vi "Configure.vi"(8 "error in (no error)":errorcluster, 11 "Waveform in":refnum<class "Waveform.lvclass">) -> (0 "error out":errorcluster, 2 "cancelled?":bool, 3 "Waveform out":refnum<class "Waveform.lvclass">)   [LabVIEW 2012, in "Waveform.lvclass"]
doc: "The configure method configures the details for the RabbitMQ connection, the observers and the mapping script.\n\nIn the derived class, make a call to the parent for setting these parameters."
uses:
  Waveform.lvclass
  <vilib>/Distrio/Murmex/Murmex/Murmex.lvclass
  <vilib>/Utility/miscctls.llb/LVPointTypeDef.ctl
panel:
  in  "button::cancel":bool
  in  "button::ok":bool
  in  "button::configure murmex":bool
  in  "Tab Control":T1(tab)
  in  "Output Terminal 2":tag="/Dev1/PFI12" caption="Output Terminal"
  in  "Counter 2":tag="Dev1/ctr0" caption="Counter"
  in  "Frequency 2":dbl caption="Frequency"
  in  "Duty cycle 2":dbl caption="Duty cycle"
  in  "Output Terminal":tag="/Dev1/PFI12"
  in  "Counter":tag="Dev1/ctr0"
  in  "Frequency":dbl
  in  "Duty cycle":dbl
  in  "Physical Channel 3":tag="Dev1/ao0" caption="Physical Channel"
  in  "min Voltage 3":dbl caption="min Voltage"
  in  "max Voltage 3":dbl caption="max Voltage"
  in  "trigger source 3":tag caption="trigger source"
  in  "trigger edge 3":i32(ring)=10280 caption="trigger edge 2" items=["Rising"=10280, "Falling"=10171]
  in  "Physical Channel 2":tag="Dev1/ao0" caption="Physical Channel"
  in  "min Voltage 2":dbl caption="min Voltage"
  in  "max Voltage 2":dbl caption="max Voltage"
  in  "trigger source 2":tag caption="trigger source"
  in  "trigger edge 2":i32(ring)=10280 items=["Rising"=10280, "Falling"=10171]
  in  "Physical Channel":tag="Dev1/ao0"
  in  "min Voltage":dbl
  in  "max Voltage":dbl
  in  "trigger source":tag
  in  "trigger edge":i32(ring)=10280 items=["Rising"=10280, "Falling"=10171]
  in  "camera 1":string
  in  "camera 2":string
  in  "camera 3":string
  # "RabbitMQ parameters"
  # "Window position"
  # "Sends a setting or configuration value to an observer, e.g. observer.parameter=settingsname;"
  # "Frame counter"
  # "Clock for AO channels"
  # "Galvo 1"
  # "Galvo 2"
  # "Pockels Cell"
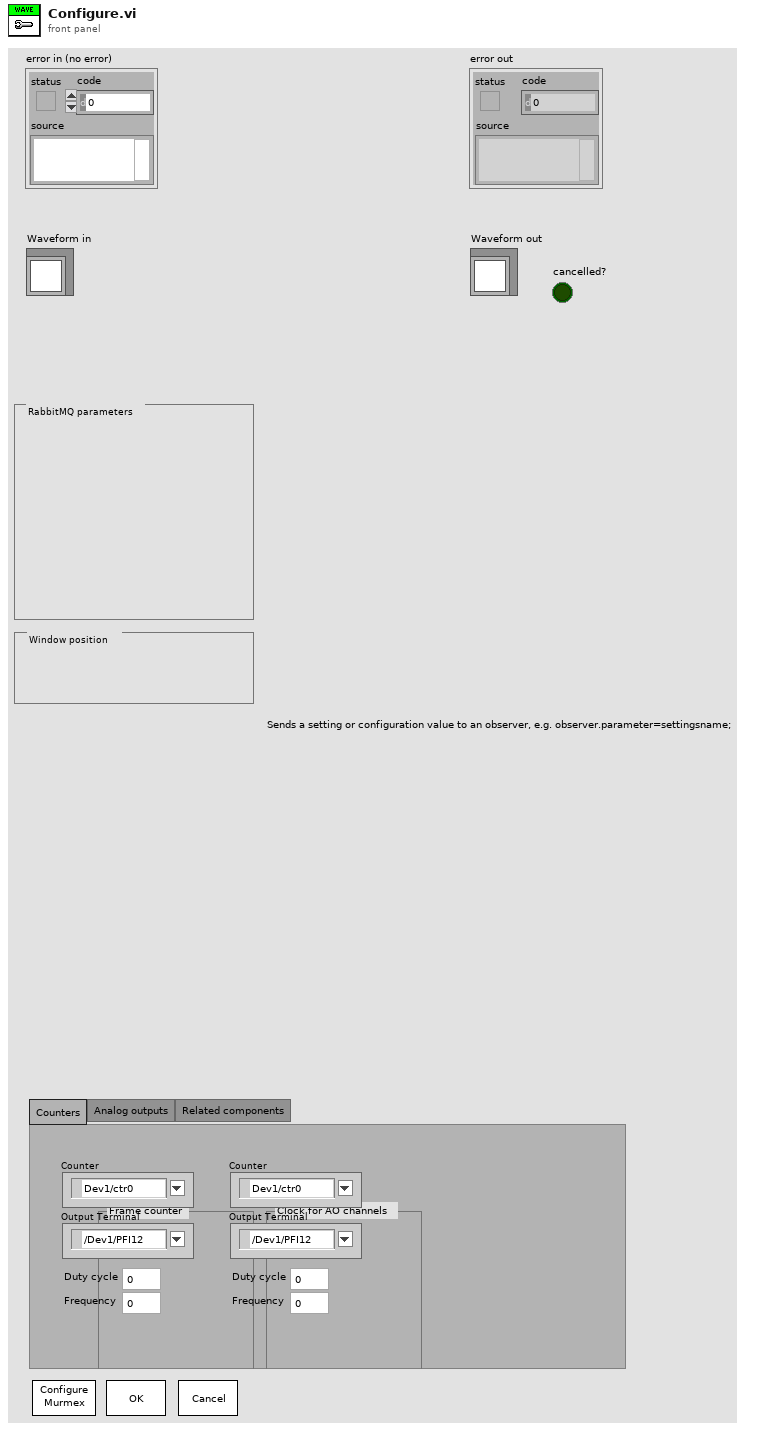
[diagram p1: front panel]
types:
  T1 = enum32{"Counters", "Analog outputs", "Related components"}
  T2 = typedef "LVPointTypeDef.ctl" = cluster{"Horizontal":i16, "Vertical":i16}
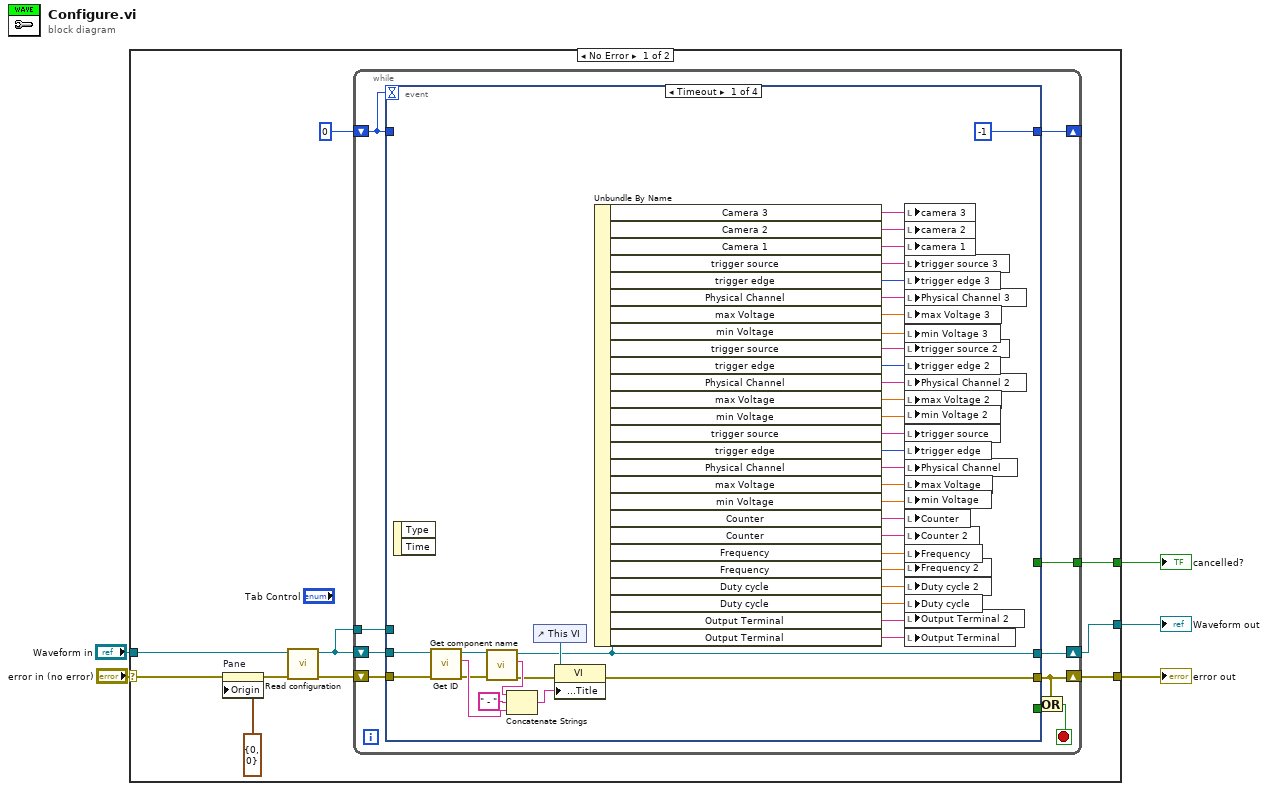
[diagram p0: block diagram]
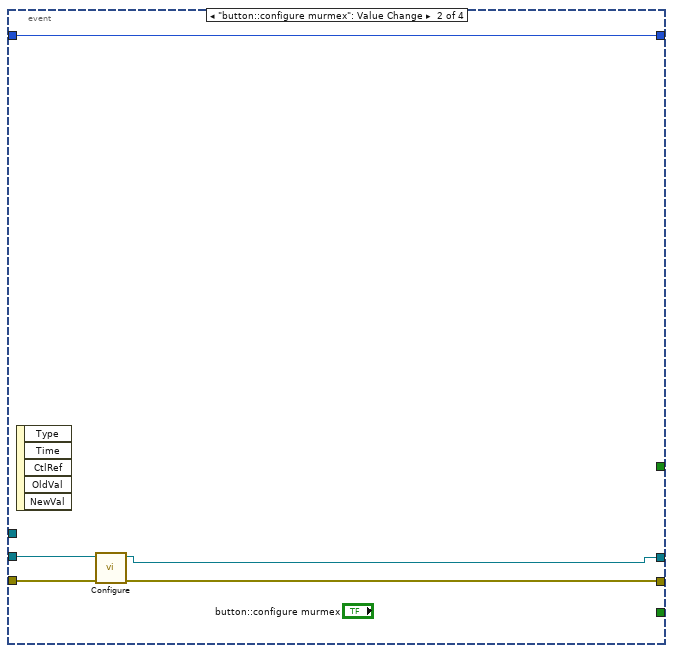
[diagram p2: hidden frame]
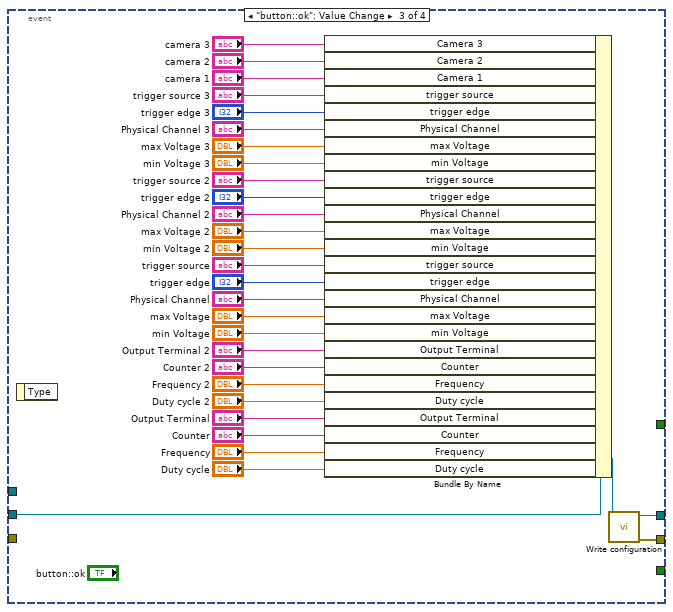
[diagram p3: hidden frame]
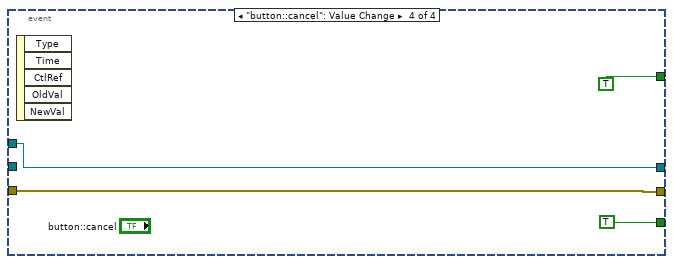
[diagram p4: hidden frame]
diagram:
  n1 = case shown="No Error" "error in (no error)" {
    selector: "error in (no error)" -> [w14 w105]
    tunnel: "Waveform in" -> [w12 w104]
    tunnel: [w8 w105] -> w3
    tunnel: [w7 w104] -> w2
    tunnel: [w6 _] -> w1
    frame No Error {
      n2 = property on="Pane" class="Pane"(error in=w14, "Origin"=T2 {"Horizontal"=0, "Vertical"=0}) -> (error out=w13:errorcluster)  [unwired: 1 in, 1 out]
      n3 = call <vilib>:"Read configuration.vi"("error in (no error)"=w13, "Murmex in"=w12) -> ("error out"=w11:errorcluster, "Murmex out"=w10:refnum<class "Waveform.lvclass">)  [unwired: 7 in, 1 out]
      n4 = while {
        shift-right: [w19] -> w8
        shift-left: w11 -> [w25]
        shift-right: [w21] -> w7
        shift-left: w10 -> [w23]
        tunnel: w10 -> [w24]
        shift-right: [w20] -> _
        shift-left: 0 -> [w22]
        tunnel: [w16] -> w6
        stop <- w18 stop-if-true
        n5 = event shown="[0] Timeout" {
          selector: _ -> [_ _ _ _]
          dyn-events: _ -> [_ _ _ _]
          timeout: w22 -> [_ _ _ _]
          tunnel: w25 -> [w64 w69 _ w103]
          tunnel: w24 -> [_ _ _ w102]
          tunnel: w23 -> [w63 w66 w97 _]
          tunnel: w22 -> [_ w67 _ _]
          tunnel: [w54 w68 w98 w103] -> w19
          tunnel: [w53 w65 w99 w102] -> w21
          tunnel: [-1 w67 _ _] -> w20
          tunnel: [_ _ _ TRUE ("force loading?")] -> w17
          tunnel: [_ _ _ TRUE ("force loading?")] -> w16
          event Timeout {
            n6 = event-data() -> ()  [unwired: 1 in, 2 out]
            n7 = call <vilib>:"Get ID.vi"("error in (no error)"=w64, "Murmex in"=w63) -> ("error out"=w58:errorcluster, "component id"=w61:string, "Murmex out"=w59:refnum<class "Waveform.lvclass">)  [unwired: 7 in]
            n8 = call <vilib>:"Get component name.vi"("error in (no error)"=w58, "Murmex in"=w59) -> ("error out"=w56:errorcluster, "component name"=w60:string, "Murmex out"=w53:refnum<class "Waveform.lvclass">)  [unwired: 7 in]
            n9 = Concatenate Strings(w60, " - " ("string"), w61) -> (w55:string)
            n10 = control-ref of="This VI"() -> (w57:refnum<vi>)
            n11 = property class="VI"(reference=w57, error in=w56, "Front Panel.Title"=w55) -> (error out=w54:errorcluster)  [unwired: 1 out]
            n12 = Unbundle By Name(w53) -> ("Camera 3"=w26:string, "Camera 2"=w27:string, "Camera 1"=w28:string, "trigger source"=w29:tag, "trigger edge"=w30:i32, "Physical Channel"=w31:tag, "max Voltage"=w32:dbl, "min Voltage"=w33:dbl, "trigger source"=w38:tag, "trigger edge"=w37:i32, "Physical Channel"=w36:tag, "max Voltage"=w35:dbl, "min Voltage"=w34:dbl, "trigger source"=w39:tag, "trigger edge"=w40:i32, "Physical Channel"=w41:tag, "max Voltage"=w42:dbl, "min Voltage"=w43:dbl, "Counter"=w46:tag, "Counter"=w47:tag, "Frequency"=w45:dbl, "Frequency"=w44:dbl, "Duty cycle"=w48:dbl, "Duty cycle"=w49:dbl, "Output Terminal"=w51:tag, "Output Terminal"=w50:tag)
            n13 = local write "camera 3"(w26) -> ()
            n14 = local write "camera 2"(w27) -> ()
            n15 = local write "camera 1"(w28) -> ()
            n16 = local write "trigger source 3"(w29) -> ()
            n17 = local write "trigger edge 3"(w30) -> ()
            n18 = local write "Physical Channel 3"(w31) -> ()
            n19 = local write "max Voltage 3"(w32) -> ()
            n20 = local write "min Voltage 3"(w33) -> ()
            n21 = local write "trigger source 2"(w38) -> ()
            n22 = local write "trigger edge 2"(w37) -> ()
            n23 = local write "Physical Channel 2"(w36) -> ()
            n24 = local write "max Voltage 2"(w35) -> ()
            n25 = local write "min Voltage 2"(w34) -> ()
            n26 = local write "trigger source"(w39) -> ()
            n27 = local write "trigger edge"(w40) -> ()
            n28 = local write "Physical Channel"(w41) -> ()
            n29 = local write "max Voltage"(w42) -> ()
            n30 = local write "min Voltage"(w43) -> ()
            n31 = local write "Counter"(w46) -> ()
            n32 = local write "Counter 2"(w47) -> ()
            n33 = local write "Frequency"(w45) -> ()
            n34 = local write "Frequency 2"(w44) -> ()
            n35 = local write "Duty cycle 2"(w48) -> ()
            n36 = local write "Duty cycle"(w49) -> ()
            n37 = local write "Output Terminal 2"(w51) -> ()
            n38 = local write "Output Terminal"(w50) -> ()
          }
          event "button::configure murmex": Value Change {
            n39 = event-data() -> ()  [unwired: 1 in, 5 out]
            n40 = call-parent "Configure.vi"("error in (no error)"=w69, "Murmex in"=w66) -> ("error out"=w68:errorcluster, "Murmex out"=w65:refnum<class "Waveform.lvclass">)  [unwired: 7 in, 1 out]
          }
          event "button::ok": Value Change {
            n41 = event-data() -> ()  [unwired: 1 in, 1 out]
            n42 = Bundle By Name(cluster=w97, "Camera 3"="camera 3", "Camera 2"="camera 2", "Camera 1"="camera 1", "trigger source"="trigger source 3", "trigger edge"="trigger edge 3", "Physical Channel"="Physical Channel 3", "max Voltage"="max Voltage 3", "min Voltage"="min Voltage 3", "trigger source"="trigger source 2", "trigger edge"="trigger edge 2", "Physical Channel"="Physical Channel 2", "max Voltage"="max Voltage 2", "min Voltage"="min Voltage 2", "trigger source"="trigger source", "trigger edge"="trigger edge", "Physical Channel"="Physical Channel", "max Voltage"="max Voltage", "min Voltage"="min Voltage", "Output Terminal"="Output Terminal 2", "Counter"="Counter 2", "Frequency"="Frequency 2", "Duty cycle"="Duty cycle 2", "Output Terminal"="Output Terminal", "Counter"="Counter", "Frequency"="Frequency", "Duty cycle"="Duty cycle") -> (w96:refnum<class "Waveform.lvclass">)
            n43 = call <vilib>:"Write configuration.vi"("Murmex in"=w96) -> ("error out"=w98:errorcluster, "Murmex out"=w99:refnum<class "Waveform.lvclass">)  [unwired: 9 in]
          }
          event "button::cancel": Value Change {
            n44 = event-data() -> ()  [unwired: 1 in, 5 out]
          }
        }
        n45 = Or(x=w19, y=w17) -> (x .or. y?=w18:bool)
      }
    }
    frame Error {
    }
  }
  "error out" <- w3
  "Waveform out" <- w2
  "cancelled?" <- w1
